vi "Motor Begin.vi"(8 "error in (no error)":errorcluster) -> (0 "error out":errorcluster)   [LabVIEW 2014]
uses:
  <vilib>/Rock Robotics/SystemInterfaces/DIO/FPGA_DIOPWMChannel.ctl
  <vilib>/Rock Robotics/WPI/MotorControl/WPI_MotorControlOpen Talon.vi
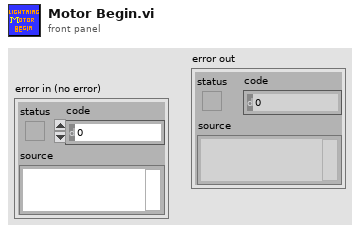
[diagram p1: front panel]
types:
  T1 = typedef "FPGA_DIOPWMChannel.ctl" = enum8{"PWM 0", "PWM 1", "PWM 2", "PWM 3", "PWM 4", "PWM 5", "PWM 6", "PWM 7", "PWM 8", "PWM 9", "PWM MXP 0", "PWM MXP 1", "PWM MXP 2", "PWM MXP 3", "PWM MXP 4", "PWM MXP 5", "PWM MXP 6", "PWM MXP 7", "PWM MXP 8", "PWM MXP 9", "Invalid"}
  T2 = typedef "WPI_MotorControlDeviceRef.ctl" = cluster{"DeviceStatus":errorcluster, "Type":T3, "PWM":cluster{"Controller":T4, "PWM Channel":T1, "DeadBand":T5}, "CAN":cluster{"Device Number":u8, "Control Mode":T6, "Semaphore":T7, "Max Vout":dbl, "TalonSRX Control Mode":T8}, "Invert":bool, "TransformRef":T9, "InvTransformRef":T9}
  T3 = typedef "WPI_MotorControlType.ctl" = enum16{"PWM", "CAN", "CANTalonSRX"}
  T4 = typedef "FPGA_TypedefDigitalModule.ctl" = enum16{"Controller 1"}
  T5 = typedef "WPI_PWMDeadband.ctl" = cluster{"Name":string, "maxPositivePwm":i32, "minPositivePwm":i32, "centerPwm":i32, "maxNegativePwm":i32, "minNegativePwm":i32, "angularRange":u16}
  T6 = typedef "WPI_CANJaguar_ControlMode.ctl" = enum8{"Percent VBus", "Current", "Speed", "Position", "Voltage"}
  T7 = typedef "Semaphore RefNum" = refnum<k1>
  T8 = typedef "WPI_CANTalonSRX_APIControlMode.ctl" = enum8{"Percent VBus", "Speed", "Position", "Slave", "Unchanged / Invalid"}
  T9 = typedef "WPI_PWMTransform_ConPane.ctl" = refnum<vi>
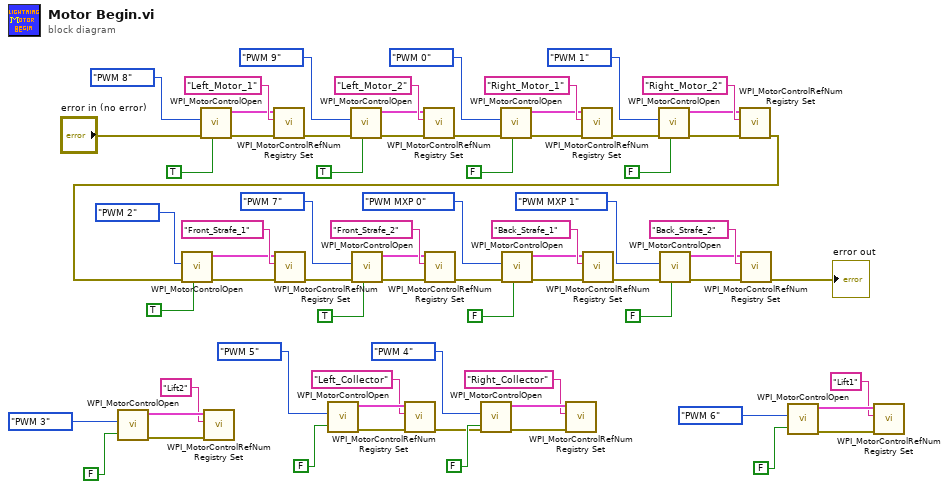
[diagram p0: block diagram]
diagram:
  n1 = call-poly <vilib>:"WPI_MotorControlOpen.vi"("Invert"=FALSE, "PWM Channel"=FPGA_DIOPWMChannel."PWM 3") -> ("error out"=w11:errorcluster, "MotorControlDeviceRef"=w12:T2)  [unwired: 8 in]
  n2 = call-poly <vilib>:"WPI_MotorControlOpen.vi"("Invert"=TRUE, "error in (no error)"="error in (no error)", "PWM Channel"=FPGA_DIOPWMChannel."PWM 8") -> ("error out"=w64:errorcluster, "MotorControlDeviceRef"=w60:T2)  [unwired: 7 in]
  n3 = call <vilib>:"WPI_MotorControlRefNum Registry Set.vi"("error in (no error)"=w11, "refnum name"="Lift2", "MotorControlDevRef"=w12) -> ()  [unwired: 7 in, 2 out]
  n4 = call <vilib>:"WPI_MotorControlRefNum Registry Set.vi"("error in (no error)"=w64, "refnum name"="Left_Motor_1", "MotorControlDevRef"=w60) -> ("error out"=w70:errorcluster)  [unwired: 7 in, 1 out]
  n5 = call-poly <vilib>:"WPI_MotorControlOpen.vi"("Invert"=FALSE, "PWM Channel"=FPGA_DIOPWMChannel."PWM 5") -> ("error out"=w20:errorcluster, "MotorControlDeviceRef"=w21:T2)  [unwired: 8 in]
  n6 = call-poly <vilib>:"WPI_MotorControlOpen.vi"("Invert"=TRUE, "error in (no error)"=w70, "PWM Channel"=FPGA_DIOPWMChannel."PWM 9") -> ("error out"=w69:errorcluster, "MotorControlDeviceRef"=w66:T2)  [unwired: 7 in]
  n7 = call <vilib>:"WPI_MotorControlRefNum Registry Set.vi"("error in (no error)"=w20, "refnum name"="Left_Collector", "MotorControlDevRef"=w21) -> ("error out"=w13:errorcluster)  [unwired: 7 in, 1 out]
  n8 = call <vilib>:"WPI_MotorControlRefNum Registry Set.vi"("error in (no error)"=w69, "refnum name"="Left_Motor_2", "MotorControlDevRef"=w66) -> ("error out"=w54:errorcluster)  [unwired: 7 in, 1 out]
  n9 = call-poly <vilib>:"WPI_MotorControlOpen.vi"("Invert"=FALSE, "error in (no error)"=w13, "PWM Channel"=FPGA_DIOPWMChannel."PWM 4") -> ("error out"=w16:errorcluster, "MotorControlDeviceRef"=w17:T2)  [unwired: 7 in]
  n10 = call-poly <vilib>:"WPI_MotorControlOpen.vi"("Invert"=FALSE, "error in (no error)"=w54, "PWM Channel"=FPGA_DIOPWMChannel."PWM 0") -> ("error out"=w55:errorcluster, "MotorControlDeviceRef"=w47:T2)  [unwired: 7 in]
  n11 = call <vilib>:"WPI_MotorControlRefNum Registry Set.vi"("error in (no error)"=w16, "refnum name"="Right_Collector", "MotorControlDevRef"=w17) -> ()  [unwired: 7 in, 2 out]
  n12 = call <vilib>:"WPI_MotorControlRefNum Registry Set.vi"("error in (no error)"=w55, "refnum name"="Right_Motor_1", "MotorControlDevRef"=w47) -> ("error out"=w49:errorcluster)  [unwired: 7 in, 1 out]
  n13 = call-poly <vilib>:"WPI_MotorControlOpen.vi"("Invert"=FALSE, "error in (no error)"=w49, "PWM Channel"=FPGA_DIOPWMChannel."PWM 1") -> ("error out"=w50:errorcluster, "MotorControlDeviceRef"=w48:T2)  [unwired: 7 in]
  n14 = call <vilib>:"WPI_MotorControlRefNum Registry Set.vi"("error in (no error)"=w50, "refnum name"="Right_Motor_2", "MotorControlDevRef"=w48) -> ("error out"=w24:errorcluster)  [unwired: 7 in, 1 out]
  n15 = call-poly <vilib>:"WPI_MotorControlOpen.vi"("Invert"=TRUE, "error in (no error)"=w24, "PWM Channel"=FPGA_DIOPWMChannel."PWM 2") -> ("error out"=w27:errorcluster, "MotorControlDeviceRef"=w25:T2)  [unwired: 7 in]
  n16 = call <vilib>:"WPI_MotorControlRefNum Registry Set.vi"("error in (no error)"=w27, "refnum name"="Front_Strafe_1", "MotorControlDevRef"=w25) -> ("error out"=w46:errorcluster)  [unwired: 7 in, 1 out]
  n17 = call-poly <vilib>:"WPI_MotorControlOpen.vi"("Invert"=TRUE, "error in (no error)"=w46, "PWM Channel"=FPGA_DIOPWMChannel."PWM 7") -> ("error out"=w45:errorcluster, "MotorControlDeviceRef"=w42:T2)  [unwired: 7 in]
  n18 = call <vilib>:"WPI_MotorControlRefNum Registry Set.vi"("error in (no error)"=w45, "refnum name"="Front_Strafe_2", "MotorControlDevRef"=w42) -> ("error out"=w36:errorcluster)  [unwired: 7 in, 1 out]
  n19 = call-poly <vilib>:"WPI_MotorControlOpen.vi"("Invert"=FALSE, "error in (no error)"=w36, "PWM Channel"=FPGA_DIOPWMChannel."PWM MXP 0") -> ("error out"=w37:errorcluster, "MotorControlDeviceRef"=w29:T2)  [unwired: 7 in]
  n20 = call <vilib>:"WPI_MotorControlRefNum Registry Set.vi"("error in (no error)"=w37, "refnum name"="Back_Strafe_1", "MotorControlDevRef"=w29) -> ("error out"=w31:errorcluster)  [unwired: 7 in, 1 out]
  n21 = call-poly <vilib>:"WPI_MotorControlOpen.vi"("Invert"=FALSE, "error in (no error)"=w31, "PWM Channel"=FPGA_DIOPWMChannel."PWM MXP 1") -> ("error out"=w32:errorcluster, "MotorControlDeviceRef"=w30:T2)  [unwired: 7 in]
  n22 = call <vilib>:"WPI_MotorControlRefNum Registry Set.vi"("error in (no error)"=w32, "refnum name"="Back_Strafe_2", "MotorControlDevRef"=w30) -> ("error out"=→"error out":errorcluster)  [unwired: 7 in, 1 out]
  n23 = call-poly <vilib>:"WPI_MotorControlOpen.vi"("Invert"=FALSE, "PWM Channel"=FPGA_DIOPWMChannel."PWM 6") -> ("error out"=w6:errorcluster, "MotorControlDeviceRef"=w7:T2)  [unwired: 8 in]
  n24 = call <vilib>:"WPI_MotorControlRefNum Registry Set.vi"("error in (no error)"=w6, "refnum name"="Lift1", "MotorControlDevRef"=w7) -> ()  [unwired: 7 in, 2 out]
